vi "FTW-TestRunner-WriteToStdOut.vi"(8 "error in (no error)":errorcluster, 10 "Output":string="test output", 11 "WindowTitle":string="ftw-testrunner") -> (0 "error out":errorcluster)   [LabVIEW 2013]
uses:
  kernel32.dll
  user32.dll
panel:
  out "return type":i32
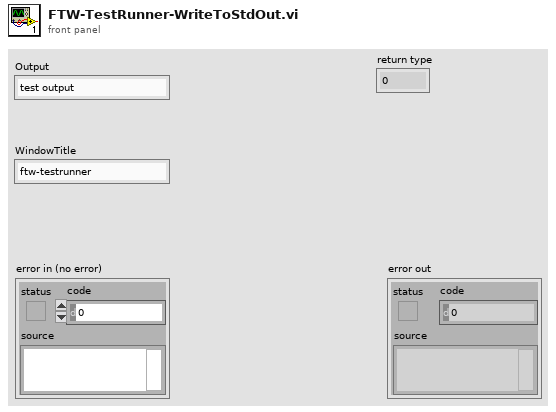
[diagram p1: front panel]
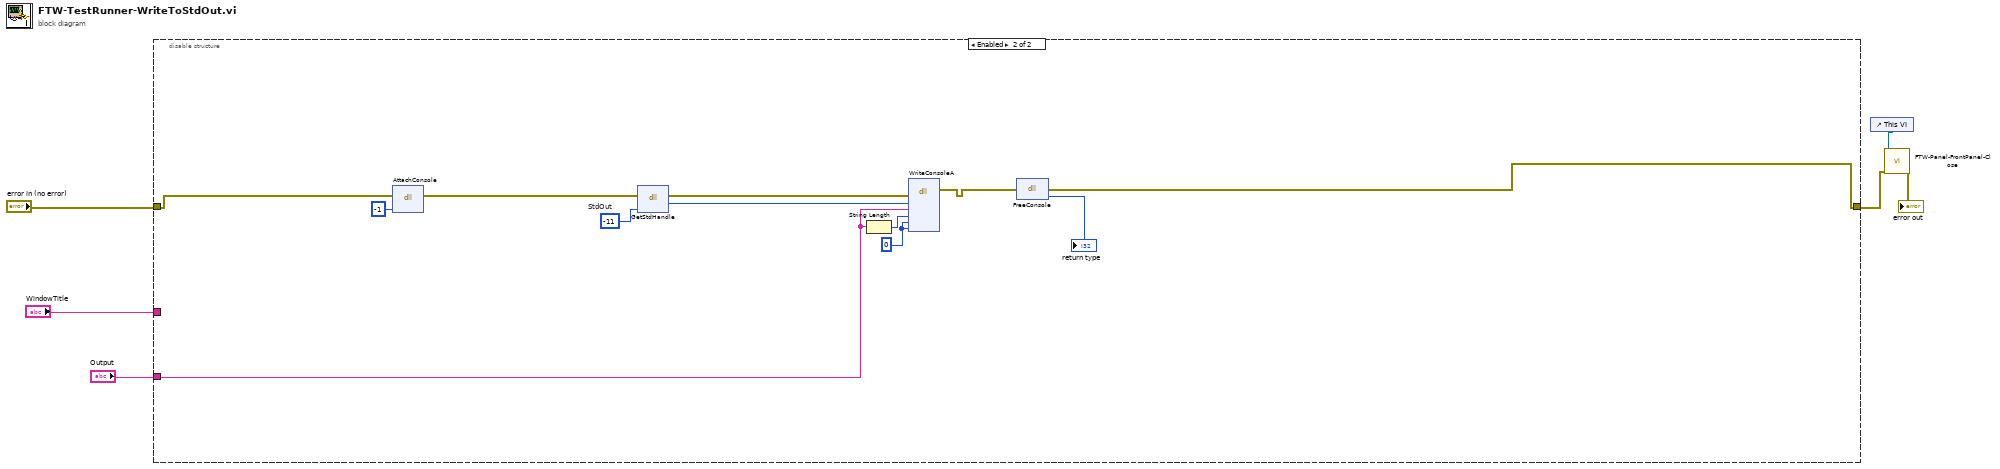
[diagram p0: block diagram]
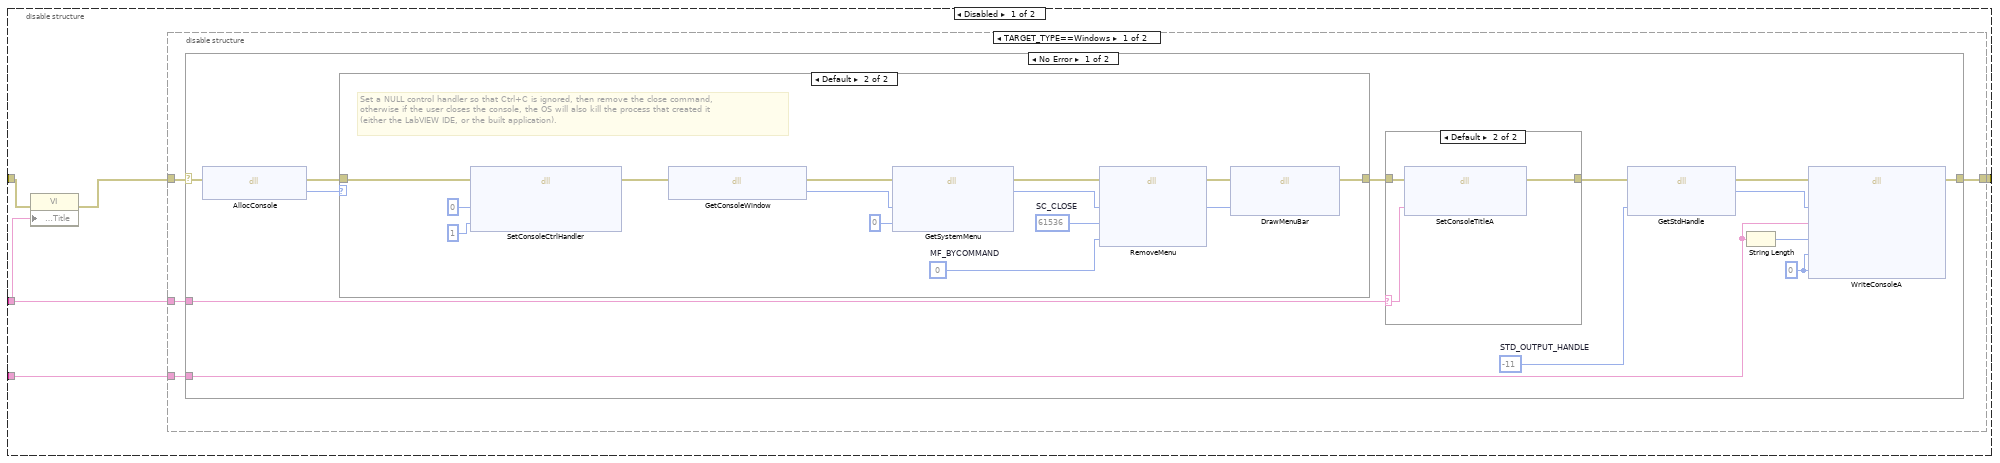
[diagram p2: hidden frame]
diagram:
  n1 = disable-structure shown="Enabled" {
    disable-tunnel: "Output" -> [w11 w52]
    disable-tunnel: [w10 w50] -> w2
    disable-tunnel: "error in (no error)" -> [w9 w51]
    disable-tunnel: "WindowTitle" -> [w7 _]
    frame Disabled {
      n2 = property class="VI"(error in=w9, "Front Panel.Title"=w7) -> (error out=w8:errorcluster)  [unwired: 1 in, 1 out]
      n3 = disable-structure shown="TARGET_TYPE==Windows" {
        disable-tunnel: w8 -> [w14 w49]
        disable-tunnel: [w15 w49] -> w10
        disable-tunnel: w7 -> [w13 _]
        disable-tunnel: w11 -> [w12 _]
        frame condition #0 (active) {
          n4 = case shown="No Error" w14 {
            selector: w14 -> [w28 w48]
            tunnel: [w17 w48] -> w15
            tunnel: w13 -> [w16 _]
            tunnel: w12 -> [w19 _]
            frame No Error {
              w21 = 0 ("lpNumberOfCharsWritten")
              w24 = -11  # STD_OUTPUT_HANDLE
              n5 = dll-call lib="kernel32.dll" fn="AllocConsole"(error in=w28) -> (error out=w26:errorcluster, "return type"=w27:i32)  [unwired: 2 in, 1 out]
              n6 = case shown="Default" w27 {
                tunnel: w26 -> [w33 w34]
                tunnel: [w33 w47] -> w25
                frame 0 {
                  # "Allocation failed, we must already have a console..."
                }
                frame Default {
                  w42 = u32 0  # MF_BYCOMMAND
                  w43 = u32 61536  # SC_CLOSE
                  # "Set a NULL control handler so that Ctrl+C is ignored, then remove the close command,\notherwise if the user closes the console, the OS will also kill the process that created it\n(either the LabVIEW IDE, or the built application)."
                  n7 = dll-call lib="kernel32.dll" fn="SetConsoleCtrlHandler"(error in=w34, "HandlerRoutine"=u32 0, "Add"=1) -> (error out=w37:errorcluster)  [unwired: 2 in, 4 out]
                  n8 = dll-call lib="kernel32.dll" fn="GetConsoleWindow"(error in=w37) -> (error out=w40:errorcluster, "return type"=w46:i32)  [unwired: 2 in, 1 out]
                  n9 = dll-call lib="user32.dll" fn="GetSystemMenu"(error in=w40, "hWnd"=w46, "bRevert"=0) -> (error out=w39:errorcluster, "return type"=w44:i32)  [unwired: 4 in, 1 out]
                  n10 = dll-call lib="user32.dll" fn="RemoveMenu"(error in=w39, "hMenu"=w44, "uPosition"=w43, "uFlags"=w42) -> (error out=w38:errorcluster, "hMenu"=w41:i32)  [unwired: 4 in, 2 out]
                  n11 = dll-call lib="user32.dll" fn="DrawMenuBar"(error in=w38, "hMenu"=w41) -> (error out=w47:errorcluster)  [unwired: 3 in, 2 out]
                }
              }
              n12 = case shown="Default" w16 {
                selector: w16 -> [_ w30]
                tunnel: w25 -> [w29 w32]
                tunnel: [w29 w31] -> w18
                frame "" {
                }
                frame Default {
                  n13 = dll-call lib="kernel32.dll" fn="SetConsoleTitleA"(error in=w32, "lpConsoleTitle"=w30) -> (error out=w31:errorcluster)  [unwired: 2 in, 3 out]
                }
              }
              n14 = dll-call lib="kernel32.dll" fn="GetStdHandle"(error in=w18, "nStdHandle"=w24) -> (error out=w23:errorcluster, "return type"=w22:i32)  [unwired: 3 in, 1 out]
              n15 = String Length(string=w19) -> (length=w20:i32)
              n16 = dll-call lib="kernel32.dll" fn="WriteConsoleA"(error in=w23, "hConsoleOutput"=w22, "lpBuffer"=w19, "numberOfCharsToWrite"=w20, "lpNumberOfCharsWritten"=w21, "lpReserved"=w21) -> (error out=w17:errorcluster)  [unwired: 5 in, 4 out]
            }
            frame Error {
            }
          }
        }
        frame condition #1 {
        }
      }
    }
    frame Enabled {
      w60 = -11  # StdOut
      w58 = 0 ("lpNumberOfCharsWritten")
      n17 = dll-call lib="kernel32.dll" fn="AttachConsole"(error in=w51, "arg1"=-1) -> (error out=w59:errorcluster)  [unwired: 4 in, 1 out]
      n18 = dll-call lib="kernel32.dll" fn="GetStdHandle"(error in=w59, "nStdHandle"=w60) -> (error out=w55:errorcluster, "return type"=w56:i32)  [unwired: 3 in, 1 out]
      n19 = String Length(string=w52) -> (length=w57:i32)
      n20 = dll-call lib="kernel32.dll" fn="WriteConsoleA"(error in=w55, "hConsoleOutput"=w56, "lpBuffer"=w52, "numberOfCharsToWrite"=w57, "lpNumberOfCharsWritten"=w58, "lpReserved"=w58) -> (error out=w54:errorcluster)  [unwired: 5 in, 4 out]
      n21 = dll-call lib="kernel32.dll" fn="FreeConsole"(error in=w54) -> (error out=w50:errorcluster, "return type"=→"return type":i32)  [unwired: 2 in, 1 out]
    }
  }
  n22 = control-ref of="This VI"() -> (w1:refnum<vi>)
  n23 = call "FTW-Panel-FrontPanel-Close.vi"("error in"=w2, "VI Ref"=w1) -> ("error out"=→"error out":errorcluster)  [unwired: 8 in, 1 out]
